vi "Shutdown System.vi"(4 "System Status":refnum<vi>, 6 "Error Queue":refnum<queue>, 8 "error in (no error)":errorcluster) -> (0 "error out":errorcluster)   [LabVIEW 2019]
uses:
  Variables/Globals/Global_Initialized.vi
panel:
  # "--- Outputs ---"
  # "--- Inputs ---"
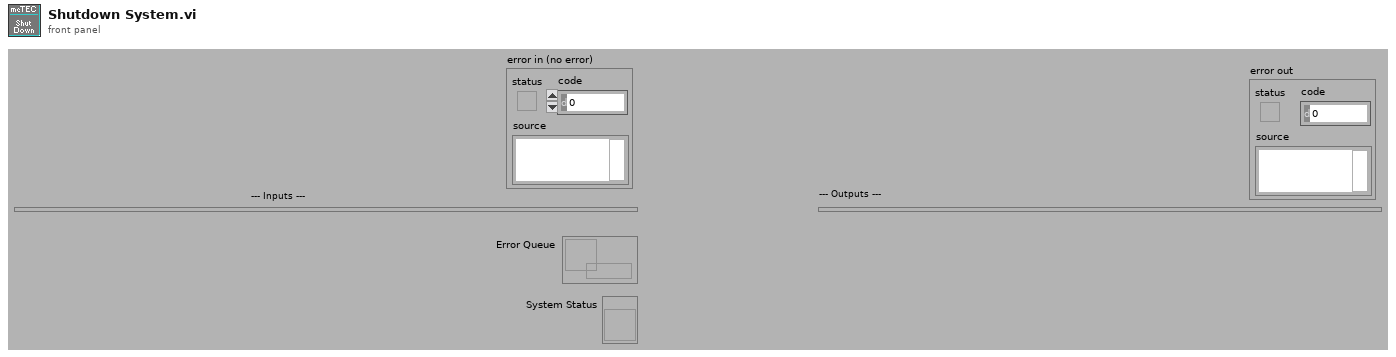
[diagram p1: front panel]
types:
  T1 = typedef "FGV_TE Controller.ctl" = cluster{"SVs":cluster{"Unused":dbl}, "PVs":cluster{"FW & HW Versions":cluster{"Device Type [I32]":i32, "Device Type [String]":string, "Firmware Version [I32]":i32, "Firmware Version [String]":string, "Hardware Version [I32]":i32, "Hardware Version [String]":string, "Serial No.":i32}, "TEC Configuration":T2, "Object Target Temperature Source_CH1":u8, "Object Target Temperature Source_CH2":u8}, "Front Panel References":T3}
  T2 = typedef "meTEC_Configuration.ctl" = cluster{"VISA resource name":refnum<visa-resource-name>, "Device Address":u16}
  T3 = typedef "FGV_Front Panel References.ctl" = cluster{"Main Loop Queue":refnum<queue>, "meTEC_Device Type":refnum<vi>, "meTEC_Serial No.":refnum<vi>, "meTEC_Hardware Version":refnum<vi>, "meTEC_Firmware Version":refnum<vi>, "meTEC_CH1_Object Target Temperature (ID 3000 / 50012) [°C]":refnum<vi>, "meTEC_CH1_Live Set Current (ID 50001) [A]":refnum<vi>, "meTEC_CH1_Live Set Voltage (ID 50002) [V]":refnum<vi>, "meTEC_CH1_Live Enable (ID 50000)":refnum<vi>, "meTEC_CH1_Input Selection (ID 2000)":refnum<vi>, "meTEC_CH1_Object Target Temp. Source Sel. (ID 50011)":refnum<vi>, "meTEC_CH2_Object Target Temperature (ID 3000 / 50012) [°C]":refnum<vi>, "meTEC_CH2_Live Set Current (ID 50001) [A]":refnum<vi>, "meTEC_CH2_Live Set Voltage (ID 50002) [V]":refnum<vi>, "meTEC_CH2_Live Enable (ID 50000)":refnum<vi>, "meTEC_CH2_Input Selection (ID 2000)":refnum<vi>, "meTEC_CH2_Object Target Temp. Source Sel. (ID 50011)":refnum<vi>, "meTEC_CH2_Object Temperature [°C]":refnum<vi>, "meTEC_CH2_Sink Temperature [°C]":refnum<vi>, "meTEC_CH2_Act. Output Current [A]":refnum<vi>, "meTEC_CH2_Act. Output Voltage [V]":refnum<vi>, "meTEC_CH2_Temperature Stability":refnum<vi>, "Monitor Chart_CH2":refnum<vi>, "meTEC_Initialize Device":refnum<vi>}
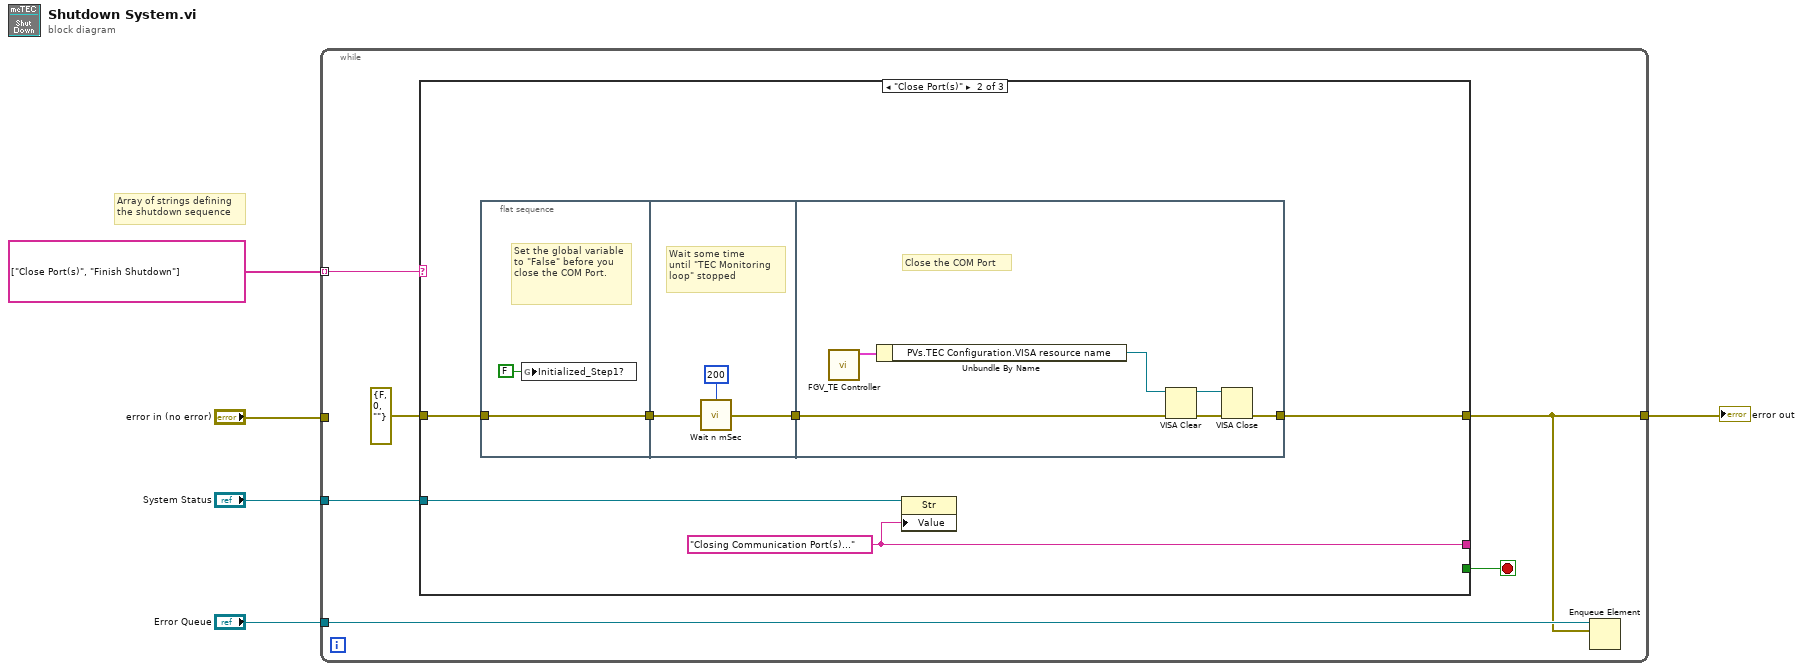
[diagram p0: block diagram]
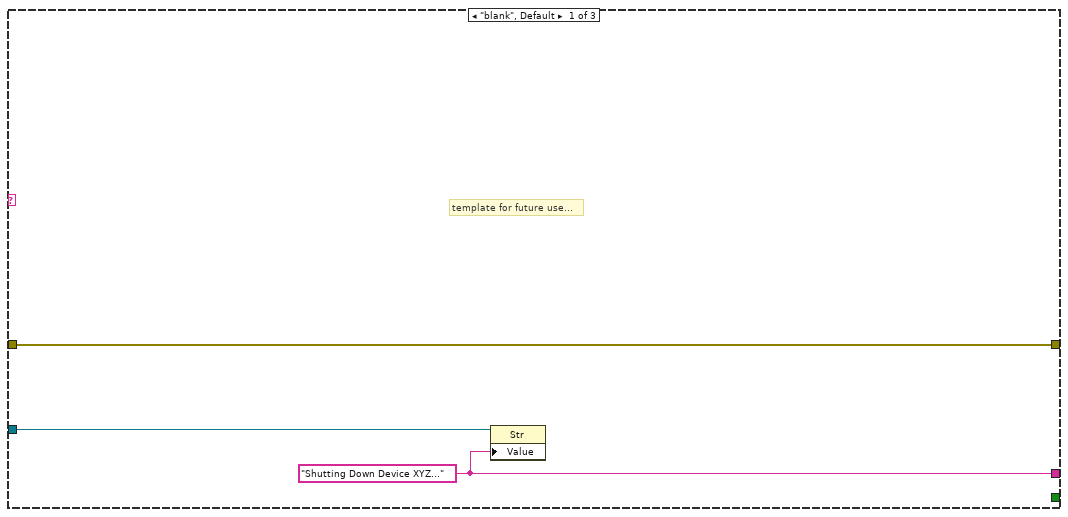
[diagram p2: hidden frame]
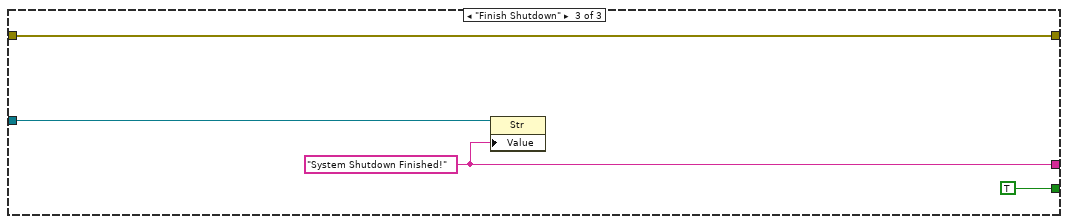
[diagram p3: hidden frame]
diagram:
  # "Array of strings defining\nthe shutdown sequence"
  n1 = while {
    tunnel: "Error Queue" -> [w11]
    tunnel: string[] ["Close Port(s)", "Finish Shutdown"] -> [w10] mode=indexing
    tunnel: "System Status" -> [w8]
    tunnel: "error in (no error)" -> [_]
    tunnel: [w6] -> w4
    stop <- w9 stop-if-true
    n2 = case shown="\"Close Port(s)\"" w10 {
      tunnel: errorcluster {"status"=FALSE, "code"=0, "source"=""} ("error in (no error)") -> [w12 w17 w33]
      tunnel: [w12 w18 w33] -> w6
      tunnel: [_ _ TRUE ("status")] -> w9
      tunnel: w8 -> [w14 w20 w34]
      tunnel: [w13 w19 w32] -> _
      frame "blank", Default {
        w13 = "Shutting Down Device XYZ..." ("Value")
        # "template for future use..."
        n3 = property class="Str"(reference=w14, "Value"=w13) -> ()  [unwired: 1 in, 2 out]
      }
      frame "Close Port(s)" {
        w19 = "Closing Communication Port(s)..." ("Value")
        n4 = flat-sequence {
          tunnel: w17 -> [w22]
          tunnel: [w22] -> w15
          tunnel: [w24] -> w16
          tunnel: w15 -> [w25]
          tunnel: [w31] -> w18
          tunnel: w16 -> [w26]
          frame #0 {
            # "Set the global variable\nto \"False\" before you\nclose the COM Port."
            n5 = global write "Global_Initialized.vi" "Initialized_Step1?"(FALSE ("Initialized?")) -> ()
          }
          frame #1 {
            # "Wait some time\nuntil \"TEC Monitoring\nloop\" stopped"
            n6 = call "Wait n mSec.vi"("error in (no error)"=w25, "milliseconds to wait (500)"=u32 200) -> ("error out"=w24:errorcluster)
          }
          frame #2 {
            # "Close the COM Port"
            n7 = call "FGV_TE Controller.vi"() -> ("FGV_TEC_OUT"=w30:T1)  [unwired: 10 in, 1 out]
            n8 = Unbundle By Name(w30) -> ("PVs.TEC Configuration.VISA resource name"=w29:refnum<visa-resource-name>)
            n9 = VISA Clear(VISA resource name=w29, error in (no error)=w26) -> (VISA resource name out=w28:refnum<visa-resource-name>, error out=w27:errorcluster)
            n10 = VISA Close(VISA resource name=w28, error in (no error)=w27) -> (error out=w31:errorcluster)
          }
        }
        n11 = property class="Str"(reference=w20, "Value"=w19) -> ()  [unwired: 1 in, 2 out]
      }
      frame "Finish Shutdown" {
        w32 = "System Shutdown Finished!" ("Value")
        n12 = property class="Str"(reference=w34, "Value"=w32) -> ()  [unwired: 1 in, 2 out]
      }
    }
    n13 = Enqueue Element(queue=w11, element=w6) -> ()  [unwired: 2 in, 3 out]
  }
  "error out" <- w4
